vi "REL.vi"(0 "System no.":i32=1 min=1 max=4 step=1, 2 "Relays to command":string[](array[string]), 3 "Relay mode":bool[](array[boolean]), 5 "error in":errorcluster) -> (19 "error out":errorcluster)   [LabVIEW 2020]
doc: "Switches relays on or off. Relay identifiers are A-H for relay board 1, I-P for relay board 2 etc."
panel:
  # "Switches relays on or off. Relay identifiers are A-H for relay board \n1, I-P for relay board 2 etc."
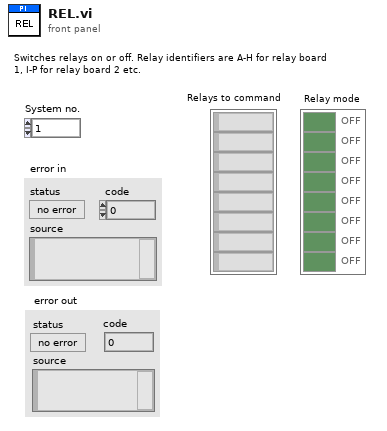
[diagram p1: front panel]
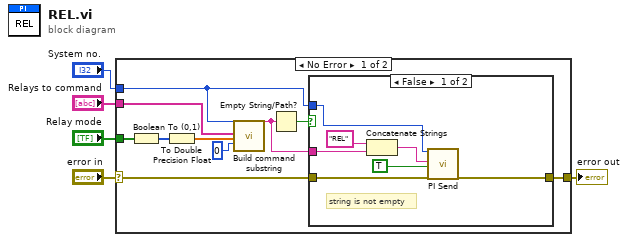
[diagram p0: block diagram]
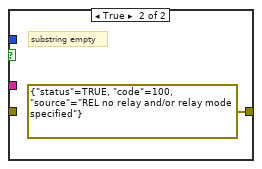
[diagram p2: hidden frame]
diagram:
  n1 = case shown="No Error" "error in" {
    selector: "error in" -> [w6 w24]
    tunnel: [w15 w24] -> w5
    tunnel: "System no." -> [w9 _]
    tunnel: "Relays to command" -> [w14 _]
    tunnel: "Relay mode" -> [w13 _]
    frame No Error {
      n2 = Boolean To (0,1)(Boolean=w13) -> (0, 1=w12:i16[])
      n3 = To Double Precision Float(number=w12) -> (double precision float=w10:dbl[])
      n4 = call "Build command substring.vi"("System no."=w9, "Affected axes"=w14, "Parameters"=w10, "No. of digits"=i16 0 ("No.of digits")) -> ("Command substring"=w7:string)  [unwired: 3 in, 12 out]
      n5 = Empty String/Path?(string/path=w7) -> (empty?=w8:bool)
      n6 = case shown="False" w8 {
        tunnel: w7 -> [w21 _]
        tunnel: [w17 errorcluster {"status"=TRUE, "code"=100, "source"="REL no relay and/or relay mode specified"} ("error out")] -> w15
        tunnel: w6 -> [w18 _]
        tunnel: w9 -> [w16 _]
        frame False {
          # "string is not empty"
          n7 = Concatenate Strings("REL", w21) -> (w19:string)
          n8 = call "PI Send.vi"("System no."=w16, "String to send"=w19, "Attach termination char.?"=TRUE ("Attach Linefeed?"), "error in"=w18) -> ("error out"=w17:errorcluster)  [unwired: 2 in, 13 out]
        }
        frame True {
          # "substring empty"
        }
      }
    }
    frame Error {
    }
  }
  "error out" <- w5
